vi "Read U16 FIFO.vi"(2 "fifo":refnum<k21>, 12 "ready for output":bool=TRUE) -> (4 "output data":u16, 10 "output valid":bool)   [LabVIEW 2011, in "FIFO.lvlib"]
uses:
  <instrlib>/RF-RIO/FIFO/FIFO/FPGA/FIFO.lvlib
  <vilib>/rvi/DataTransferAndStorage/Container/Common/niFpgaContainerExecOnDevCompGetState.vi
  <vilib>/rvi/FIFO/Fifo_Resource/nirvififoEmulationSetSize.vi
  <vilib>/rvi/DataTransferAndStorage/Container/Common/niFpgaContainerGetUniqueNameForEmu.vi
  <vilib>/rvi/interface/RandomDataEmulation/nirviRandomDataFPGAFIFO.vi
  <vilib>/rvi/interface/RandomDataEmulation/niFpgaRandomDataHandleErrors.vi
  <vilib>/rvi/eio/common/nirviEmuReportErrorAndStop.vi
  <vilib>/rvi/DataTransferAndStorage/Container/XNode/niFpgaContainer.xnode
  <vilib>/rvi/FIFO/Fifo_Resource/niFpgaFifoEmulationRefIn.vi
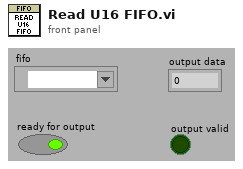
[diagram p1: front panel]
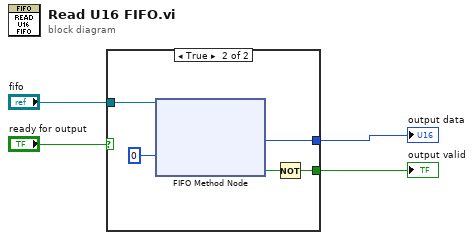
[diagram p0: block diagram]
diagram:
  n1 = case shown="True" "ready for output" {
    tunnel: "fifo" -> [_ w8]
    tunnel: [_ w6] -> w3
    tunnel: [_ w9] -> w2
    frame False {
    }
    frame True {
      n2 = xnode ("FIFO Method Node")("Timeout"=0, "FIFO In"=w8) -> ("Element"=w6:u16, "Timed Out?"=w5:bool)  [unwired: 1 out]
      n3 = Not(x=w5) -> (.not. x?=w9:bool)
    }
  }
  "output data" <- w3
  "output valid" <- w2
